vi "Polygon Intersection_Rm Duplicated Vertices.vi"(9 "tolerance":dbl=1e-10, 10 "Y":dbl[](array[numeric]), 11 "X":dbl[](array[numeric])) -> (2 "Y out":dbl[](array[numeric]), 3 "X out":dbl[](array[numeric]))   [LabVIEW 2017, in "NI_AAL_Geometry.lvlib"]
uses:
  <vilib>/Analysis/NI_AAL_Geometry.lvlib
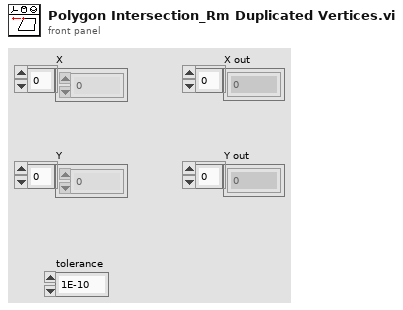
[diagram p1: front panel]
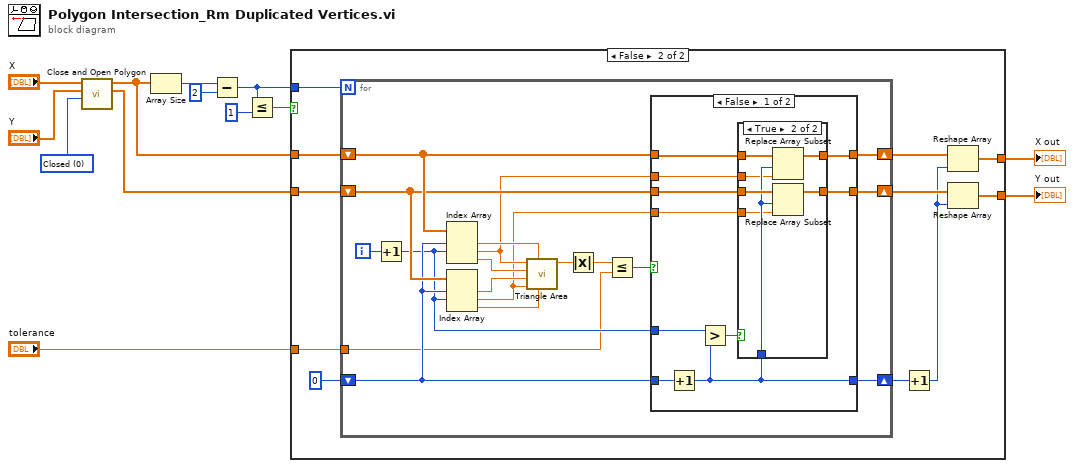
[diagram p0: block diagram]
diagram:
  w1 = u16 0 items=["Closed", "Open"] ("type")
  n1 = call <vilib>:"Close and Open Polygon.vi"("type"=w1, "Y In"="Y", "X In"="X") -> ("Y Out"=w2:dbl[], "X Out"=w4:dbl[])  [unwired: 7 in]
  n2 = Array Size(array=w4) -> (size(s)=w7:i32)
  n3 = Subtract(x=w7, y=2) -> (x-y=w11:i32)
  n4 = Less Or Equal?(x=w11, y=1) -> (x <= y?=w12:bool)
  n5 = case shown="False" w12 {
    tunnel: w4 -> [w15 w25]
    tunnel: w2 -> [w14 w24]
    tunnel: "tolerance" -> [_ w23]
    tunnel: w11 -> [_ w18]
    tunnel: [w15 w17] -> w9
    tunnel: [w14 w16] -> w8
    frame True {
    }
    frame False {
      n6 = for {
        N: w18 -> [_]
        shift-right: [w43] -> w22
        shift-left: w25 -> [w44]
        shift-right: [w42] -> w21
        shift-left: w24 -> [w40]
        tunnel: w23 -> [w36]
        shift-right: [w41] -> w20
        shift-left: 0 -> [w38]
        i -> [w39]
        n7 = Increment(x=w39) -> (x+1=w37:i32)
        n8 = Index Array(array=w44, index #1=w38, index #2=w37) -> (element #1=w32:dbl, element #2=w31:dbl, element #3=w30:dbl)  [unwired: 1 in]
        n9 = Index Array(array=w40, index #1=w38, index #2=w37) -> (element #1=w29:dbl, element #2=w28:dbl, element #3=w27:dbl)  [unwired: 1 in]
        n10 = call <vilib>:"Triangle Area.vi"("y 3"=w27, "x 1"=w32, "y 2"=w28, "y 1"=w29, "x 3"=w30, "x 2"=w31) -> ("area"=w35:dbl)  [unwired: 5 in]
        n11 = Absolute Value(x=w35) -> (abs(x)=w33:dbl)
        n12 = Less Or Equal?(x=w33, y=w36) -> (x <= y?=w34:bool)
        n13 = case shown="False" w34 {
          tunnel: w44 -> [w54 w66]
          tunnel: w40 -> [w52 w65]
          tunnel: [w53 w66] -> w43
          tunnel: [w51 w65] -> w42
          tunnel: w38 -> [w46 w64]
          tunnel: [w45 w64] -> w41
          tunnel: w37 -> [w49 _]
          tunnel: w31 -> [w48 _]
          tunnel: w28 -> [w47 _]
          frame False {
            n14 = Increment(x=w46) -> (x+1=w45:i32)
            n15 = Greater?(x=w49, y=w45) -> (0:w50:bool)
            n16 = case shown="True" w50 {
              tunnel: w54 -> [w56 w63]
              tunnel: [w56 w62] -> w53
              tunnel: w45 -> [_ w59]
              tunnel: w52 -> [w55 w61]
              tunnel: [w55 w60] -> w51
              tunnel: w48 -> [_ w58]
              tunnel: w47 -> [_ w57]
              frame False {
              }
              frame True {
                n17 = Replace Array Subset(array=w63, new element=w58, index=w59) -> (w62:dbl[])
                n18 = Replace Array Subset(array=w61, new element=w57, index=w59) -> (w60:dbl[])
              }
            }
          }
          frame True {
          }
        }
      }
      n19 = Increment(x=w20) -> (x+1=w19:i32)
      n20 = Reshape Array(w22, w19) -> (w17:dbl[])
      n21 = Reshape Array(w21, w19) -> (w16:dbl[])
    }
  }
  "X out" <- w9
  "Y out" <- w8
